vi "Close.vi"(8 "error in (no error)":errorcluster, 11 "Reference in":T1={"Device"="", "Function"="", "delay"=20}) -> (0 "error out":errorcluster)   [LabVIEW 2021, in "Rigol DM3052.lvlib"]
uses:
  Rigol DM3052.lvlib
  Reference.ctl
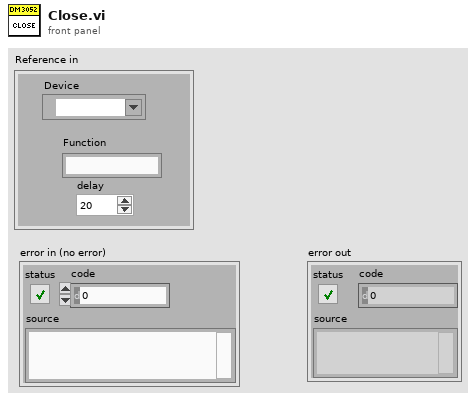
[diagram p1: front panel]
types:
  T1 = typedef "Rigol DM3052.lvlib/Reference.ctl" = cluster{"Device":refnum<visa-resource-name>, "Function":string, "delay":u32}
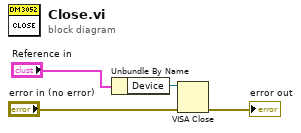
[diagram p0: block diagram]
diagram:
  n1 = Unbundle By Name("Reference in") -> ("Device"=w1:refnum<visa-resource-name>)
  n2 = VISA Close(VISA resource name=w1, error in (no error)="error in (no error)") -> (error out=→"error out":errorcluster)
